vi "Write.vi"(8 "error in (no error)":errorcluster caption="entrée d'erreur (pas d'erreur)", 11 "Class UART (Default) en entrée":refnum<class "Class UART P2056.lvclass">) -> (0 "error out":errorcluster caption="sortie d'erreur", 3 "Class UART (Default) en sortie":refnum<class "Class UART P2056.lvclass">)   [LabVIEW 2020, in "Library Instrument & Equipement.lvlib" / "Library UART.lvlib" / "Class UART P2056.lvclass"]
uses:
  Class UART P2056.lvclass
  UART (Default)/Class UART (Default).lvclass
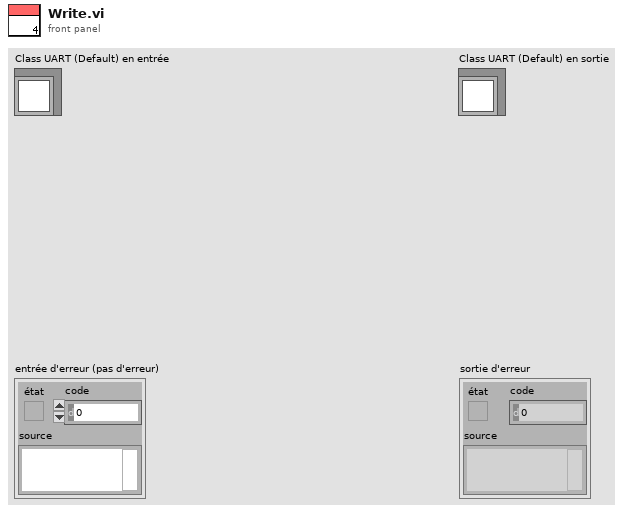
[diagram p1: front panel]
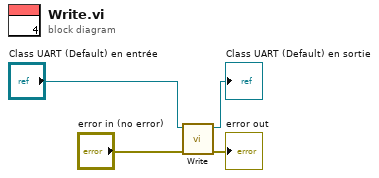
[diagram p0: block diagram]
diagram:
  n1 = call-parent "Write.vi"("error in (no error)"="error in (no error)", "Class UART (Default) en entrée"="Class UART (Default) en entrée") -> ("error out"=→"error out":errorcluster, "Class UART (Default) en sortie"=→"Class UART (Default) en sortie":refnum<class "Class UART P2056.lvclass">)  [unwired: 8 in]
